vi "Position to XML.vi"(8 "error in (no error)":errorcluster, 11 "StageSPIM in":refnum<class "StageSPIM.lvclass">) -> (0 "error out":errorcluster, 2 "XML string":string, 3 "StageSPIM out":refnum<class "StageSPIM.lvclass">)   [LabVIEW 2012, in "StageSPIM.lvclass"]
uses:
  StageSPIM.lvclass
  StageSPIM.lvclass/StageSPIM.ctl
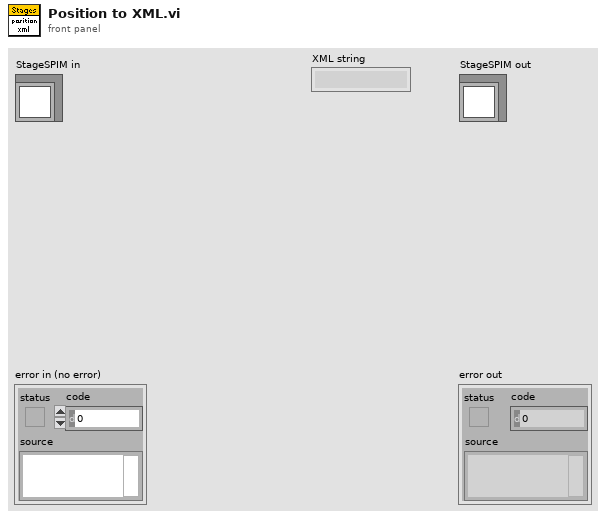
[diagram p1: front panel]
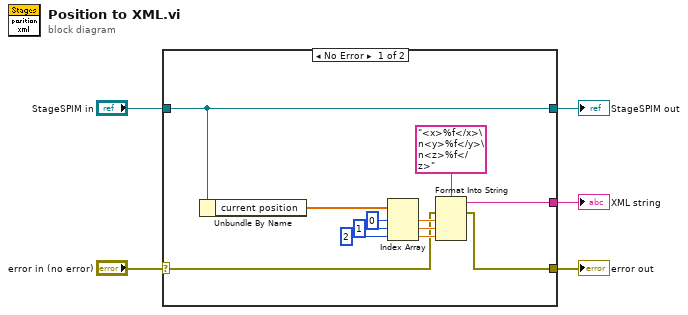
[diagram p0: block diagram]
diagram:
  n1 = case shown="No Error" "error in (no error)" {
    selector: "error in (no error)" -> [w8 w19]
    tunnel: [w7 w19] -> w4
    tunnel: [w17 w18] -> w2
    tunnel: "StageSPIM in" -> [w17 w18]
    tunnel: [w6 _] -> w1
    frame No Error {
      n2 = Unbundle By Name(w17) -> ("current position"=w16:dbl[])
      n3 = Index Array(array=w16, index #1=0 ("index"), index #2=1 ("index"), index #3=2 ("index")) -> (element #1=w11:dbl, element #2=w10:dbl, element #3=w9:dbl)
      n4 = Format Into String(format string="<x>%f</x>\n<y>%f</y>\n<z>%f</z>", error in=w8, w11, w10, w9) -> (resulting string=w6:string, error out=w7:errorcluster)  [unwired: 1 in]
    }
    frame Error {
    }
  }
  "error out" <- w4
  "StageSPIM out" <- w2
  "XML string" <- w1
